vi "Step_SetPosition.vi"(6 "Position":dbl, 7 "device_reference":i32, 8 "error in (no error)":errorcluster, 10 "Settings":T1, 11 "WindmillDevice in":refnum<class "WindmillDevice.lvclass">) -> (0 "error out":errorcluster, 3 "WindmillDevice out":refnum<class "WindmillDevice.lvclass">)   [LabVIEW 2020, in "WindmillDevice.lvclass"]
uses:
  WindmillDevice.lvclass
  settingsArcus_TypDef.ctl
  source/Device Drivers/shared/numericVariable_TypeDef.ctl
  WindmillDevice.lvclass/WindmillDevice.ctl
  source/Device Drivers/BaseDriver/BaseDriver.lvclass
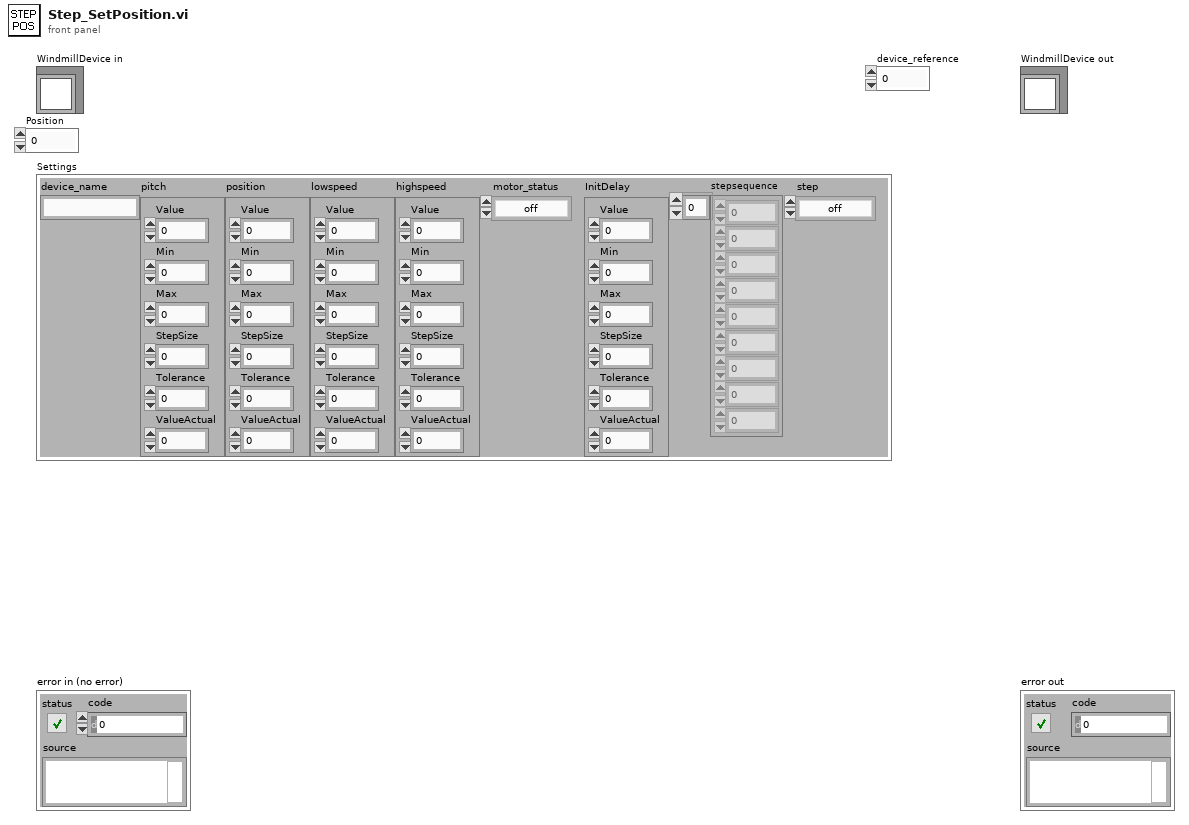
[diagram p1: front panel]
types:
  T1 = typedef "WindmillDevice.lvclass/settingsArcus_TypDef.ctl" = cluster{"device_name":string, "pitch":T2, "position":T2, "lowspeed":T2, "highspeed":T2, "motor_status":enum16{"off", "on"}, "InitDelay":T2, "stepsequence":dbl[], "step":enum16{"off", "on"}}
  T2 = typedef "BaseDriver.lvclass/numericVariable_TypeDef.ctl" = cluster{"Value":dbl, "Min":dbl, "Max":dbl, "StepSize":dbl, "Tolerance":dbl, "ValueActual":dbl}
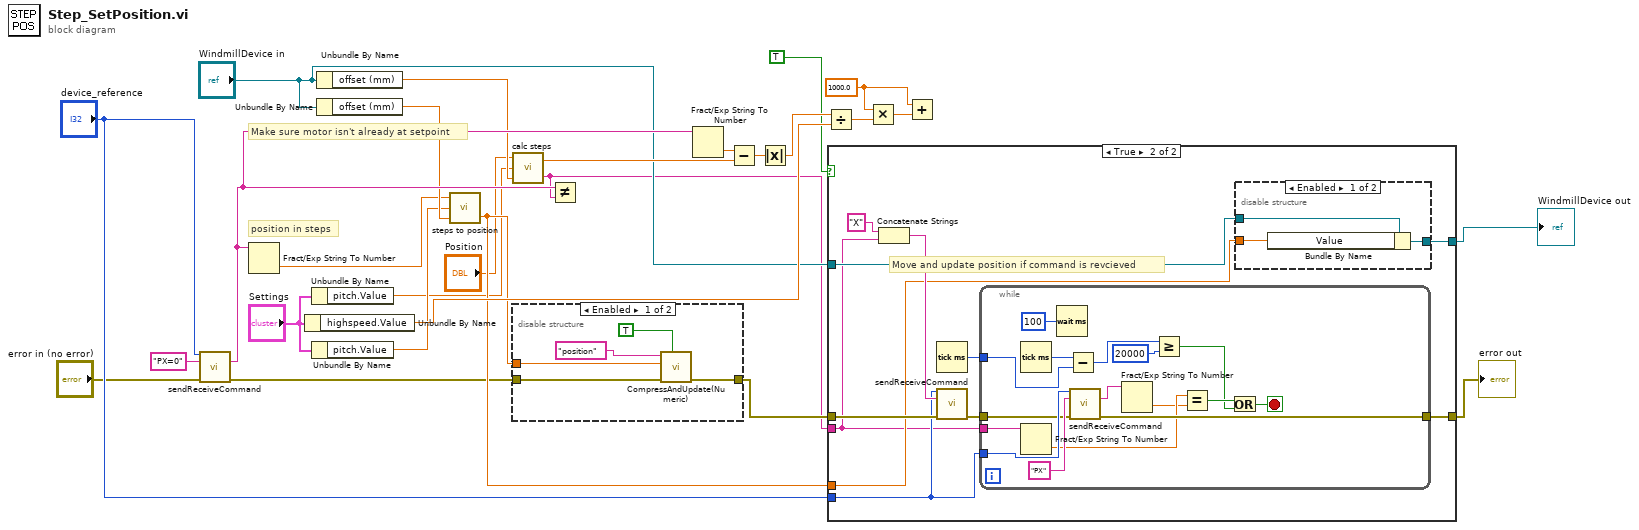
[diagram p0: block diagram]
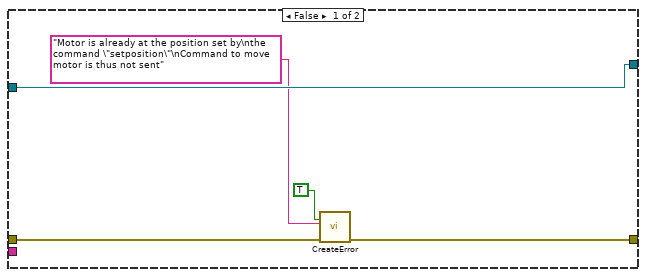
[diagram p3: hidden frame]
diagram:
  w27 = 1000.0 ("x")
  # "position in steps"
  # "Make sure motor isn't already at setpoint"
  n1 = call "sendReceiveCommand.vi"("reference (in)"="device_reference", "write_string"="PX=0", "error in (no error)"="error in (no error)") -> ("read_string"=w19:string, "error out"=w10:errorcluster)  [unwired: 10 in, 1 out]
  n2 = Fract/Exp String To Number(string=w19) -> (number=w13:dbl)  [unwired: 3 in, 1 out]
  n3 = Unbundle By Name("Settings") -> ("highspeed.Value"=w23:dbl)
  n4 = Unbundle By Name("Settings") -> ("pitch.Value"=w8:dbl)
  n5 = Unbundle By Name("Settings") -> ("pitch.Value"=w14:dbl)
  n6 = Unbundle By Name("WindmillDevice in") -> ("offset (mm)"=w9:dbl)
  n7 = Unbundle By Name("WindmillDevice in") -> ("offset (mm)"=w15:dbl)
  n8 = call "steps to position.vi"("Offset (mm)"=w15, "Pitch"=w14, "position (steps)"=w13) -> ("Position  (mm)"=w17:dbl)  [unwired: 1 in]
  n9 = call "calc steps.vi"("Offset (mm)"=w9, "Pitch"=w8, "Position to set (mm)"="Position") -> ("# counts"=w2:string, "pos to set (steps)"=w21:dbl)
  n10 = disable-structure shown="Enabled" {
    disable-tunnel: w10 -> [w31 _]
    disable-tunnel: [w30 _] -> w11
    disable-tunnel: w17 -> [w29 _]
    frame Enabled {
      n11 = call "CompressAndUpdate(Numeric).vi"("force CVT update (false)"=TRUE, "error in"=w31, "Numeric"=w29, "command or variable name"="position") -> ("error out"=w30:errorcluster)  [unwired: 7 in]
    }
    frame Disabled {
    }
  }
  n12 = Not Equal?(x=w19, y=w2) -> ()  [unwired: 1 out]
  n13 = Fract/Exp String To Number(string=w19) -> (number=w20:dbl)  [unwired: 3 in, 1 out]
  n14 = Subtract(x=w20, y=w21) -> (x-y=w22:dbl)
  n15 = Absolute Value(x=w22) -> (abs(x)=w26:dbl)
  n16 = Divide(x=w26, y=w23) -> (x/y=w24:dbl)
  n17 = case shown="True" TRUE {
    tunnel: "device_reference" -> [_ w42]
    tunnel: w2 -> [_ w39]
    tunnel: w11 -> [w36 w46]
    tunnel: "WindmillDevice in" -> [w37 w45]
    tunnel: w17 -> [_ w44]
    tunnel: [w35 w40] -> w6
    tunnel: [w37 w43] -> w7
    frame False {
      n18 = call "CreateError.vi"("Warning"=TRUE, "user error in"=w36, "error message (\"\")"="Motor is already at the position set by\nthe command \"setposition\"\nCommand to move motor is thus not sent" ("error message (\"\")")) -> ("user error  out"=w35:errorcluster)  [unwired: 8 in]
    }
    frame True {
      # "Move and update position if command is revcieved"
      n19 = Concatenate Strings("X" ("raw_cmd"), w39) -> (w47:string)
      n20 = Tick Count (ms)() -> (millisecond timer value=w38:u32)
      n21 = call "sendReceiveCommand.vi"("reference (in)"=w42, "write_string"=w47, "error in (no error)"=w46) -> ("error out"=w41:errorcluster)  [unwired: 10 in, 2 out]
      n22 = while {
        tunnel: w42 -> [w63]
        tunnel: w41 -> [w61]
        tunnel: [w60] -> w40
        tunnel: w39 -> [w52]
        tunnel: w38 -> [w56]
        stop <- w58 stop-if-true
        n23 = Tick Count (ms)() -> (millisecond timer value=w57:u32)
        n24 = Fract/Exp String To Number(string=w52) -> (number=w50:dbl)  [unwired: 3 in, 1 out]
        n25 = Wait (ms)(milliseconds to wait=u32 100) -> ()  [unwired: 1 out]
        n26 = Subtract(x=w57, y=w56) -> (x-y=w55:u32)
        n27 = call "sendReceiveCommand.vi"("reference (in)"=w63, "write_string"="PX", "error in (no error)"=w61) -> ("read_string"=w51:string, "error out"=w60:errorcluster)  [unwired: 10 in, 1 out]
        n28 = Fract/Exp String To Number(string=w51) -> (number=w49:dbl)  [unwired: 3 in, 1 out]
        n29 = Greater Or Equal?(x=w55, y=u32 20000) -> (x >= y?=w53:bool)
        n30 = Equal?(x=w50, y=w49) -> (x = y?=w59:bool)
        n31 = Or(x=w59, y=w53) -> (x .or. y?=w58:bool)
      }
      n32 = disable-structure shown="Enabled" {
        disable-tunnel: w45 -> [w67 w68]
        disable-tunnel: w44 -> [w66 _]
        disable-tunnel: [w65 w68] -> w43
        frame Enabled {
          n33 = Bundle By Name(cluster=w67, "Value"=w66) -> (w65:refnum<class "WindmillDevice.lvclass">)
        }
        frame Disabled {
        }
      }
    }
  }
  "WindmillDevice out" <- w7
  "error out" <- w6
  n34 = Multiply(x=w27, y=w24) -> (x*y=w25:dbl)
  n35 = Add(x=w27, y=w25) -> ()  [unwired: 1 out]
